vi "DSF.Shared.Configuration.Transfer.Channels to Blocks.vi"(8 "error in (no error)":errorcluster, 10 "Channel Parameters":T2[](array[typedef]) {"Channel Ref" format="%016x"; "offset" format="%d bytes"}, 11 "Transfer Configuration in":refnum<class "DSF.Shared.Configuration.Transfer.lvclass">) -> (0 "error out":errorcluster, 2 "Channel Blocks":T1[](array[typedef]) {"count" format="%d elements"; "Base Channel"."Channel Ref" format="%016x"; "Base Channel"."offset" format="%d bytes"}, 3 "Transfer Configuration out":refnum<class "DSF.Shared.Configuration.Transfer.lvclass">)   [LabVIEW 2016, in "DSF.Shared.lvlib" / "DSF.Shared.Configuration.Transfer.lvclass"]
uses:
  DSF.Shared.Configuration.Transfer.lvclass
  Typedefs/DSF.Shared.Typedefs.Configuration.Transfer.Channel Parameters.ctl
  Typedefs/DSF.Shared.Typedefs.Data Type.ctl
  <vilib>/NI Veristand/Custom Device API/Custom Device Item Ref.ctl
  Typedefs/DSF.Shared.Typedefs.Configuration.Transfer.Channel Block.ctl
  DSF.Shared.lvlib
  <vilib>/NI Veristand/Custom Device API/Custom Device API.lvlib
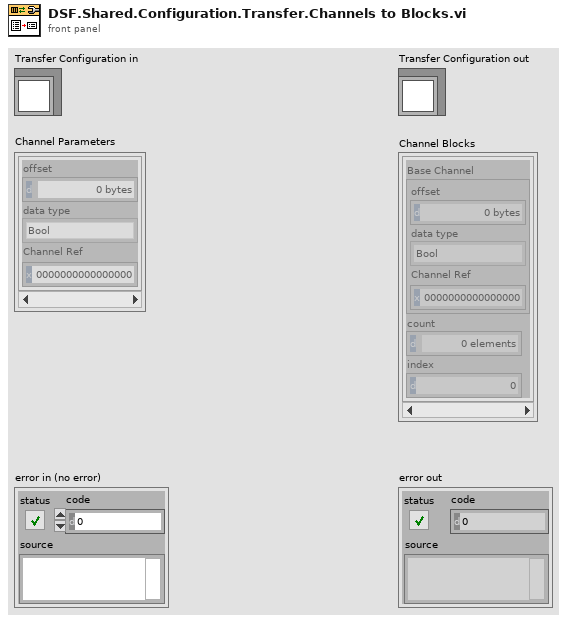
[diagram p1: front panel]
types:
  T1 = typedef "DSF.Shared.lvlib/DSF.Shared.Typedefs.Configuration.Transfer.Channel Block.ctl" = cluster{"Base Channel":T2, "count":u64, "index":u64}
  T2 = typedef "DSF.Shared.lvlib/DSF.Shared.Typedefs.Configuration.Transfer.Channel Parameters.ctl" = cluster{"offset":u64, "data type":T3, "Channel Ref":T4}
  T3 = typedef "DSF.Shared.lvlib/DSF.Shared.Typedefs.Data Type.ctl" = enum8{"Bool", "SGL", "DBL", "I8", "I16", "I32", "I64", "U8", "U16", "U32", "U64"}
  T4 = typedef "Custom Device API.lvlib/Custom Device Item Ref.ctl" = u64
  T5 = cluster{"offset":bool, "data type":bool, "Channel Ref":bool}
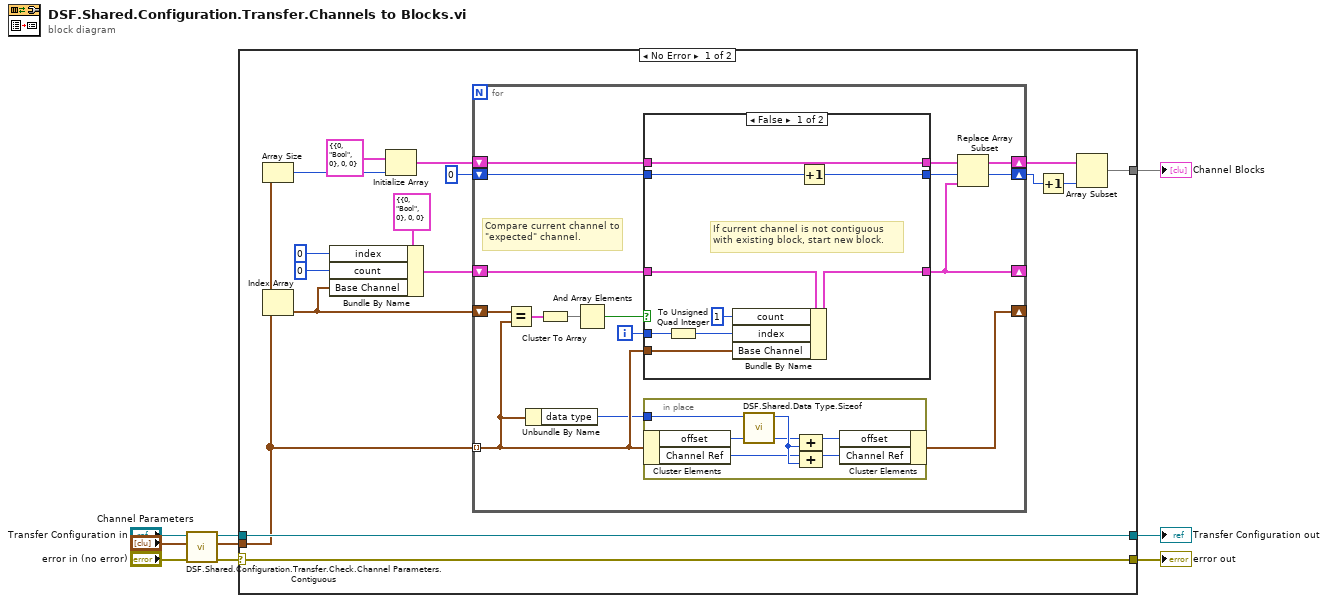
[diagram p0: block diagram]
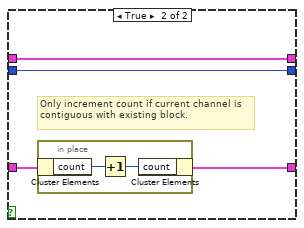
[diagram p2: hidden frame]
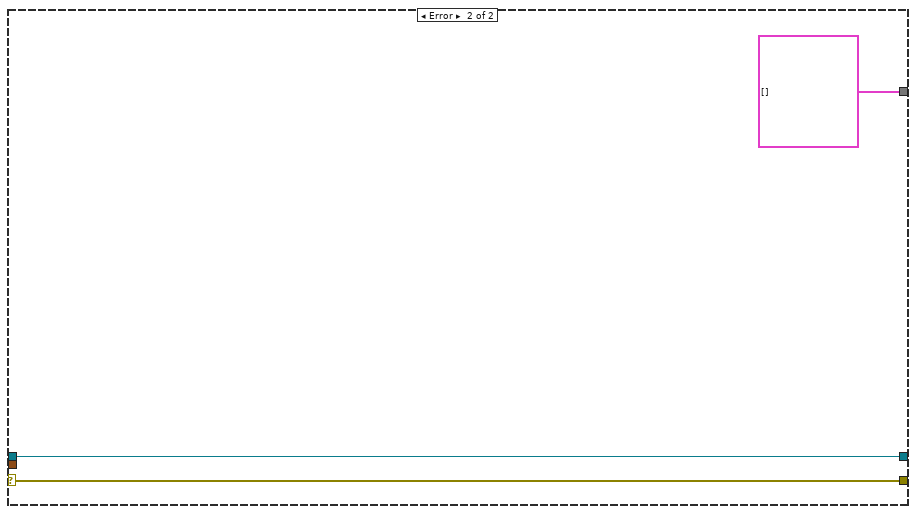
[diagram p3: hidden frame]
diagram:
  n1 = call "DSF.Shared.Configuration.Transfer.Check.Channel Parameters.Contiguous.vi"("error in (no error)"="error in (no error)", "Channels in"="Channel Parameters", "Transfer Configuration in"="Transfer Configuration in") -> ("error out"=w4:errorcluster, "Channels out"=w6:T2[], "Transfer Configuration out"=w2:refnum<class "DSF.Shared.Configuration.Transfer.lvclass">)  [unwired: 6 in]
  n2 = case shown="No Error" w4 {
    selector: w4 -> [w12 w64]
    tunnel: [w19 T1[] []] -> w9
    tunnel: w6 -> [w10 _]
    tunnel: [w12 w64] -> w3
    tunnel: w2 -> [w11 w63]
    tunnel: [w11 w63] -> w1
    frame No Error {
      n3 = Array Size(array=w10) -> (size(s)=w24:i32)
      n4 = Index Array(array=w10) -> (element=w17:T2)  [unwired: 1 in]
      n5 = Bundle By Name(cluster=T1 {"Base Channel"={"offset"=0, "data type"=enum."Bool", "Channel Ref"=0}, "count"=0, "index"=0} ("Channel Parameters"), "index"=u64 0, "count"=u64 0, "Base Channel"=w17) -> (w16:T1)
      n6 = Initialize Array(T1 {"Base Channel"={"offset"=0, "data type"=enum."Bool", "Channel Ref"=0}, "count"=0, "index"=0} ("Channel Parameters"), w24) -> (w23:T1[])
      n7 = for {
        tunnel: w10 -> [w40] mode=indexing
        shift-right: [w30] -> _
        shift-left: w17 -> [w37]
        shift-right: [w33] -> w21
        shift-left: w23 -> [w36]
        shift-right: [w32] -> w20
        shift-left: 0 ("size(s)") -> [w35]
        shift-right: [w31] -> _
        shift-left: w16 -> [w27]
        i -> [w26]
        # "Compare current channel to \"expected\" channel."
        n8 = Equal?(x=w37, y=w40) -> (x = y?=w39:T5)
        n9 = Unbundle By Name(w40) -> ("data type"=w29:T3)
        n10 = Cluster To Array(cluster=w39) -> (array=w38:bool[])
        n11 = And Array Elements(Boolean array=w38) -> (logical AND=w28:bool)
        n12 = case shown="False" w28 {
          tunnel: w27 -> [w53 w59]
          tunnel: [w52 w58] -> w31
          tunnel: w36 -> [w54 w57]
          tunnel: w35 -> [w55 w56]
          tunnel: [w51 w56] -> w32
          tunnel: [w54 w57] -> w34
          tunnel: w40 -> [w50 _]
          tunnel: w26 -> [w49 _]
          frame False {
            # "If current channel is not contiguous with existing block, start new block."
            n13 = To Unsigned Quad Integer(1:w49) -> (0:w47:u64)
            n14 = Bundle By Name(cluster=w53, "count"=u64 1, "index"=w47, "Base Channel"=w50) -> (w52:T1)
            n15 = Increment(x=w55) -> (x+1=w51:i32)
          }
          frame True {
            # "Only increment count if current channel is contiguous with existing block."
            n16 = in-place {
              n17 = in-place-cluster #1(w59) -> ("count"=w61:u64)
              n18 = Increment(x=w61) -> (x+1=w60:u64)
              n19 = in-place-cluster #1("count"=w60) -> (w58:T1)
            }
          }
        }
        n20 = in-place {
          in-place-border: w29 -> [w41]
          n21 = in-place-cluster #2(w40) -> ("offset"=w44:u64, "Channel Ref"=w45:T4)
          n22 = call "DSF.Shared.Data Type.Sizeof.vi"("data type"=w41) -> ("size in bytes"=w46:u64)  [unwired: 9 in, 1 out]
          n23 = Compound Arithmetic op=ADD(w44, w46) -> (w43:u64)
          n24 = Compound Arithmetic op=ADD(w45, w46) -> (w42:T4)
          n25 = in-place-cluster #2("offset"=w43, "Channel Ref"=w42) -> (w30:T2)
        }
        n26 = Replace Array Subset(array=w34, new element=w31, index=w32) -> (w33:T1[])
      }
      n27 = Increment(x=w20) -> (x+1=w14:i32)
      n28 = Array Subset(array=w21, length=w14) -> (w19:T1[])  [unwired: 1 in]
    }
    frame Error {
    }
  }
  "Channel Blocks" <- w9
  "error out" <- w3
  "Transfer Configuration out" <- w1
